vi "getProtocolLevel.vi"(11 "MQTTVersion50 in":refnum<class "MQTTVersion50.lvclass">) -> (2 "Protocol Level":u8 format="%08b", 3 "MQTTVersion50 out":refnum<class "MQTTVersion50.lvclass">)   [LabVIEW 2013, in "MQTT_Control_Packets_50.lvlib" / "MQTTVersion50.lvclass"]
uses:
  MQTTVersion50.lvclass
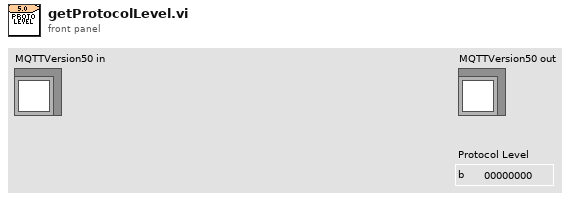
[diagram p1: front panel]
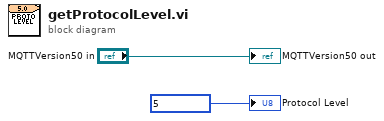
[diagram p0: block diagram]
diagram:
  "MQTTVersion50 out" <- "MQTTVersion50 in"
  "Protocol Level" <- u8 5 ("Byte")
